vi "Build Control Setting.vi"(8 "error in (no error)":errorcluster, 11 "Control Builder in":refnum<class "GUI Control Builder.lvclass">) -> (0 "error out":errorcluster, 3 "Control Builder out":refnum<class "GUI Control Builder.lvclass">)   [LabVIEW 2015, in "GUI Control Builder.lvclass"]
uses:
  GUI Control Builder.lvclass
  GUI Control Builder.lvclass/GUI Control Builder.ctl
  GUI Controls/GUI Control/GUI Control.lvclass
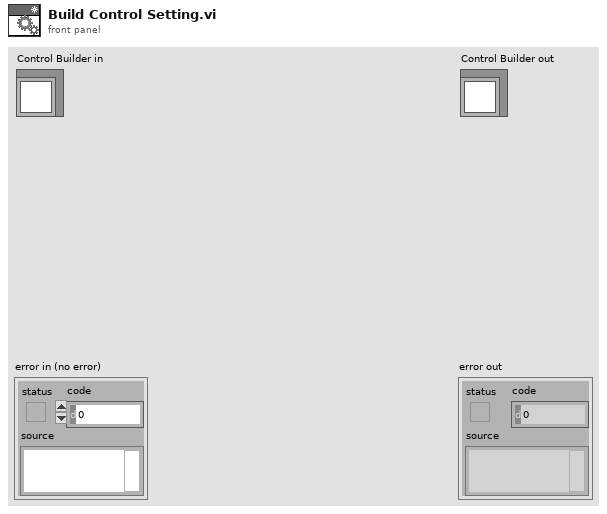
[diagram p1: front panel]
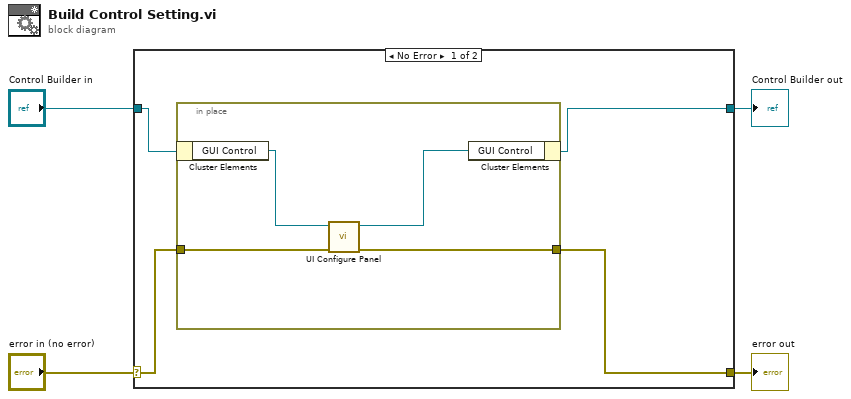
[diagram p0: block diagram]
diagram:
  n1 = case shown="No Error" "error in (no error)" {
    selector: "error in (no error)" -> [w8 w14]
    tunnel: [w7 w14] -> w3
    tunnel: [w5 w13] -> w1
    tunnel: "Control Builder in" -> [w6 w13]
    frame No Error {
      n2 = in-place {
        in-place-border: w8 -> [w12]
        in-place-border: [w11] -> w7
        n3 = in-place-cluster #1(w6) -> ("GUI Control"=w10:refnum<class "GUI Control.lvclass">)
        n4 = call-dynamic "UI Configure Panel.vi"("error in (no error)"=w12, "GUI Control in"=w10) -> ("error out"=w11:errorcluster, "GUI Control out"=w9:refnum<class "GUI Control.lvclass">)  [unwired: 8 in]
        n5 = in-place-cluster #1("GUI Control"=w9) -> (w5:refnum<class "GUI Control Builder.lvclass">)
      }
    }
    frame Error {
    }
  }
  "error out" <- w3
  "Control Builder out" <- w1
